vi "compress returns.vi"(1 "result string 2":string) -> (0 "result string":string)   [LabVIEW 2018]
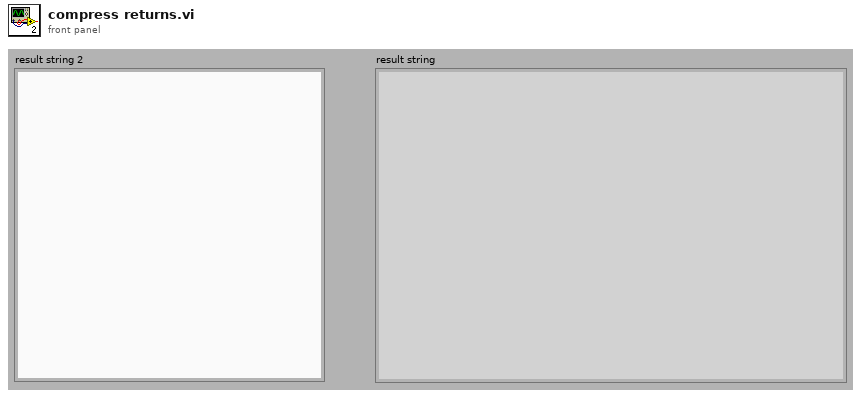
[diagram p1: front panel]
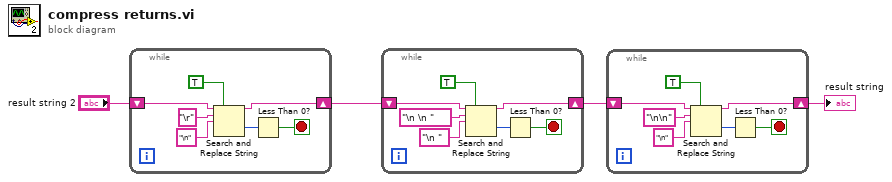
[diagram p0: block diagram]
diagram:
  n1 = while {
    shift-right: [w7] -> w2
    shift-left: "result string 2" -> [w10]
    stop <- w11 stop-if-true
    n2 = Search and Replace String(replace all?=TRUE ("replace all? (F)"), input string=w10, search string="\r", replace string="\n" ("search string")) -> (result string=w7:string, offset past replacement=w6:i32)  [unwired: 4 in, 2 out]
    n3 = Less Than 0?(x=w6) -> (x < 0?=w11:bool)
  }
  n4 = while {
    shift-right: [w14] -> w1
    shift-left: w2 -> [w17]
    stop <- w18 stop-if-true
    n5 = Search and Replace String(replace all?=TRUE ("replace all? (F)"), input string=w17, search string="\n \n ", replace string="\n " ("search string")) -> (result string=w14:string, offset past replacement=w13:i32)  [unwired: 4 in, 2 out]
    n6 = Less Than 0?(x=w13) -> (x < 0?=w18:bool)
  }
  n7 = while {
    shift-right: [w21] -> w3
    shift-left: w1 -> [w24]
    stop <- w25 stop-if-true
    n8 = Search and Replace String(replace all?=TRUE ("replace all? (F)"), input string=w24, search string="\n\n", replace string="\n" ("search string")) -> (result string=w21:string, offset past replacement=w20:i32)  [unwired: 4 in, 2 out]
    n9 = Less Than 0?(x=w20) -> (x < 0?=w25:bool)
  }
  "result string" <- w3
